vi "Error Query Global.vi"(2 "new error query setting":bool, 3 "mode (0:read value)":u16(ring) items=["read value", "set value", "remove address", "initialize globals"], 4 "GPIB address":string) -> (0 "current setting":bool, 1 "address already present?":bool)   [LabVIEW 2024]
panel:
  # "yes\nno"
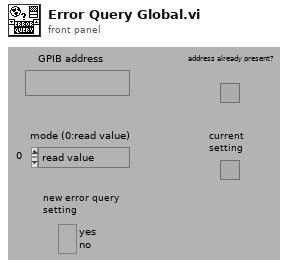
[diagram p1: front panel]
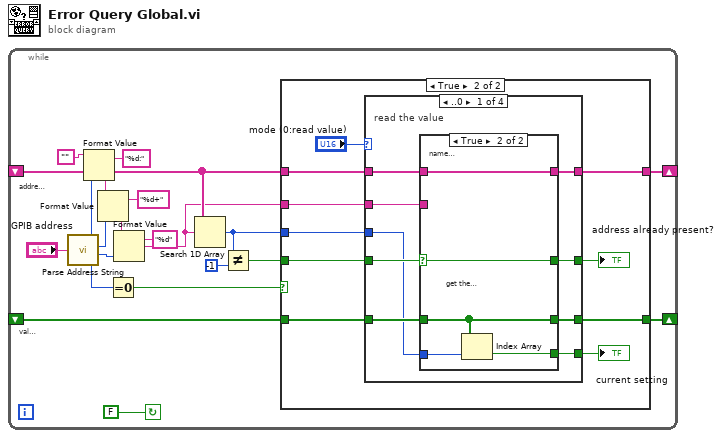
[diagram p0: block diagram]
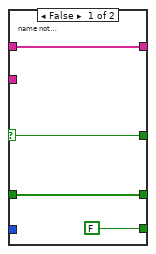
[diagram p3: hidden frame]
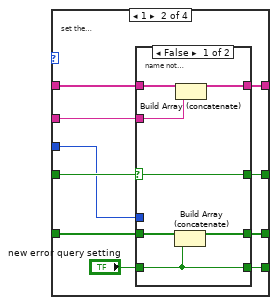
[diagram p4: hidden frame]
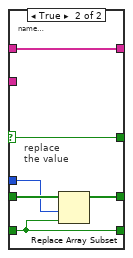
[diagram p5: hidden frame]
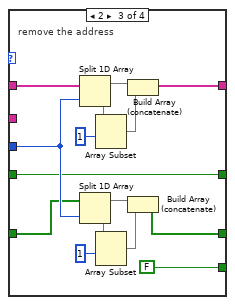
[diagram p6: hidden frame]
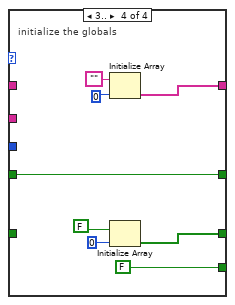
[diagram p7: hidden frame]
diagram:
  n1 = while {
    shift-right: [w8] -> _
    shift-left: _ -> [w7]
    shift-right: [w10] -> _
    shift-left: _ -> [w11]
    stop <- FALSE continue-if-true
    # "values"
    # "addresses"
    n2 = call <vilib>:"Parse Address String.vi"("address string"="GPIB address") -> ("unit"=w13:i32, "pad"=w19:i32, "sad"=w20:i32, "error"=w9:i32)
    n3 = Format Value(string ("")="", format string="%d:", value (0)=w13) -> (output string=w17:string)
    n4 = Format Value(string ("")=w17, format string="%d+", value (0)=w19) -> (output string=w18:string)
    n5 = Equal To 0?(x=w9) -> (x = 0?=w2:bool)
    n6 = Format Value(string ("")=w18, format string="%d", value (0)=w20) -> (output string=w5:string)
    n7 = Search 1D Array(1D array=w7, element=w5) -> (index of element=w4:i32)  [unwired: 1 in]
    n8 = Not Equal?(x=w4, y=-1) -> (x != y?=w3:bool)
    n9 = case shown="True" w2 {
      tunnel: w7 -> [w23 w30]
      tunnel: [w23 w31] -> w8
      tunnel: w5 -> [_ w29]
      tunnel: w11 -> [w22 w28]
      tunnel: [w22 w27] -> w10
      tunnel: w3 -> [_ w26]
      tunnel: w4 -> [_ w25]
      frame False {
      }
      frame True {
        n10 = case shown="..0" "mode (0:read value)" {
          tunnel: w30 -> [w42 w61 w85 _]
          tunnel: w28 -> [w40 w59 w77 _]
          tunnel: [w41 w60 w84 w93] -> w31
          tunnel: [w39 w58 w78 w91] -> w27
          tunnel: w29 -> [w38 w57 _ _]
          tunnel: [w37 w55 FALSE FALSE] -> w33
          tunnel: w26 -> [w36 w56 w75 w90]
          tunnel: w25 -> [w35 w53 w79 _]
          tunnel: [w34 w52 w75 w90] -> w24
          frame ..0 {
            # "read the value"
            n11 = case shown="True" w36 {
              selector: w36 -> [w43 w47]
              tunnel: w42 -> [w46 w51]
              tunnel: [w46 w51] -> w41
              tunnel: w40 -> [w45 w50]
              tunnel: [w45 w50] -> w39
              tunnel: w38 -> [_ _]
              tunnel: [FALSE w48] -> w37
              tunnel: w35 -> [_ w49]
              tunnel: [w43 w47] -> w34
              frame False {
                # "name not found"
              }
              frame True {
                # "get the value"
                # "name found"
                n12 = Index Array(array=w50, index=w49) -> (element=w48:bool)
              }
            }
          }
          frame 1 {
            # "set the value"
            n13 = case shown="False" w56 {
              selector: w56 -> [w62 w69]
              tunnel: w61 -> [w68 w74]
              tunnel: [w67 w74] -> w60
              tunnel: w59 -> [w65 w73]
              tunnel: [w64 w72] -> w58
              tunnel: "new error query setting" -> [w63 w71]
              tunnel: w57 -> [w66 _]
              tunnel: w53 -> [_ w70]
              tunnel: [w63 w71] -> w55
              tunnel: [w62 w69] -> w52
              frame False {
                # "name not found"
                n14 = Build Array (concatenate)(w65, w63) -> (w64:bool[])
                n15 = Build Array (concatenate)(w68, w66) -> (w67:string[])
              }
              frame True {
                # "replace the value"
                # "name found"
                n16 = Replace Array Subset(array=w73, new element=w71, index=w70) -> (w72:bool[])
              }
            }
          }
          frame 2 {
            # "remove the address"
            n17 = Split 1D Array(array=w85, index=w79) -> (first subarray=w88:string[], second subarray=w89:string[])
            n18 = Split 1D Array(array=w77, index=w79) -> (first subarray=w81:bool[], second subarray=w80:bool[])
            n19 = Array Subset(array=w89, index=1) -> (w87:string[])  [unwired: 1 in]
            n20 = Array Subset(array=w80, index=1) -> (w82:bool[])  [unwired: 1 in]
            n21 = Build Array (concatenate)(w88, w87) -> (w84:string[])
            n22 = Build Array (concatenate)(w81, w82) -> (w78:bool[])
          }
          frame 3.. {
            # "initialize the globals"
            n23 = Initialize Array("", 0) -> (w93:string[])
            n24 = Initialize Array(FALSE, 0) -> (w91:bool[])
          }
        }
        "current setting" <- w33
        "address already present?" <- w24
      }
    }
  }
